vi "Get_DefaultTargetDirectory.vi"(8 "error in (no error)":errorcluster, 11 "AB_Deploy_EXE in":refnum<class "AB_Deploy_EXE.lvclass">) -> (0 "error out":errorcluster, 2 "default target directory":path, 3 "AB_Deploy_EXE out":refnum<class "AB_Deploy_EXE.lvclass">)   [LabVIEW 2020, in "AB_Deploy_EXE.lvclass"]
uses:
  <vilib>/AppBuilder/AB_Classes/DeployableEXE/AB_Deploy_EXE.lvclass
  <vilib>/AppBuilder/AB_Classes/DeployableEXE/AB_Deploy_EXE.lvclass/AB_Deploy_EXE.ctl
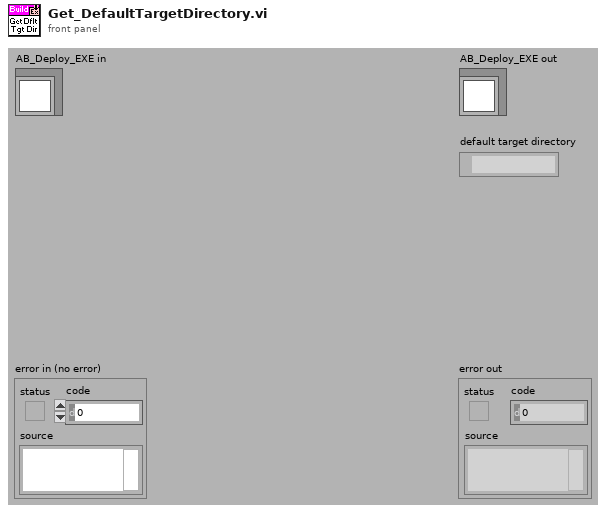
[diagram p1: front panel]
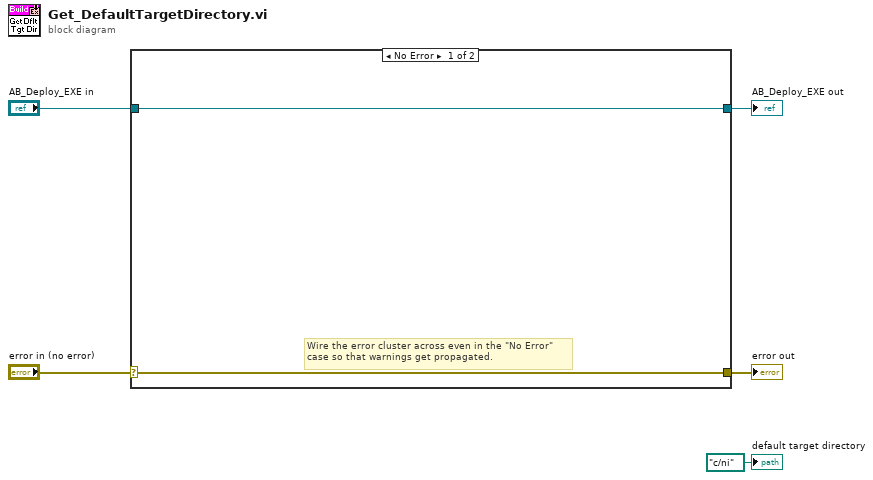
[diagram p0: block diagram]
diagram:
  n1 = case shown="No Error" "error in (no error)" {
    selector: "error in (no error)" -> [w6 w9]
    tunnel: [w6 w9] -> w4
    tunnel: [w7 w8] -> w2
    tunnel: "AB_Deploy_EXE in" -> [w7 w8]
    frame No Error {
      # "Wire the error cluster across even in the \"No Error\"\ncase so that warnings get propagated."
    }
    frame Error {
    }
  }
  "error out" <- w4
  "AB_Deploy_EXE out" <- w2
  "default target directory" <- path "c:/ni" ("default target directory")
